vi "SlingPosition.vi"(9 "PhoenixMotorControlDevRef":T1={"DeviceStatus"={"status"=FALSE, "code"=0, "source"=""}, "Type"=enum."PWM", "PWM"={"PWM Channel"=enum."PWM 1", "DeadBand"={"Name"="", "maxPositivePwm"=0, "minPositivePwm"=0, "centerPwm"=0, "maxNegativePwm"=0, "minNegativePwm"=0, "angularRange"=0}}, "CAN"={"Device Number"=0, "SetOutput VI Ref"=variant(enum8{"Percent VBus", "Current", "Speed", "Position", "Voltage"} enum."Percent VBus"), "GetOutput VI Ref"=variant(refnum<k1> refnum), "Enable VI Ref"=variant(dbl 12.0), "Disable VI Ref"=variant(enum8{"Percent VBus", "Speed", "Position", "Slave", "Unchanged / Invalid", "Voltage Compensation", "Current", "Motion Profile"} enum."Percent VBus"), "Data"=variant}, "Invert"=FALSE, "DIO PWM"={"PWM \"Enable\" Channel"=enum."Invalid", "DIOChannel"=enum."Invalid", "PWM Rate"=0.0}}, 11 "SonarSRF04DevRef":T6={"DevStatus"={"status"=FALSE, "code"=0, "source"=""}, "Ping Channel"=enum."Invalid", "Echo Channel"=enum."Invalid", "CntIndex"=enum."Invalid"}) -> (2 "Ready":bool)   [LabVIEW 2017]
uses:
  <vilib>/Rock Robotics/WPI/Ultrasonic/WPI_UltrasonicDeviceRef.ctl
  <vilib>/Rock Robotics/SystemInterfaces/DIO/FPGA_DIOChannel.ctl
  <vilib>/Rock Robotics/SystemInterfaces/Counter/FPGA_CounterCtrSystemIndex.ctl
  <vilib>/Rock Robotics/WPI/MotorControl/WPI_MotorControlDeviceRef.ctl
  <vilib>/Rock Robotics/WPI/MotorControl/WPI_MotorControlType.ctl
  <vilib>/Rock Robotics/SystemInterfaces/DIO/FPGA_DIOPWMChannel.ctl
  <vilib>/Rock Robotics/WPI/PWM/WPI_PWMDeadband.ctl
  Public/Documents/Cross The Road Electronics/Phoenix-LabVIEW/Motor Controller/Controls/CTRE_Phoenix_MotorControl_ControlMode.ctl
  <vilib>/Rock Robotics/WPI/Ultrasonic/WPI_SonarSRF04DigitalGetRange.vi
  Global 1.vi
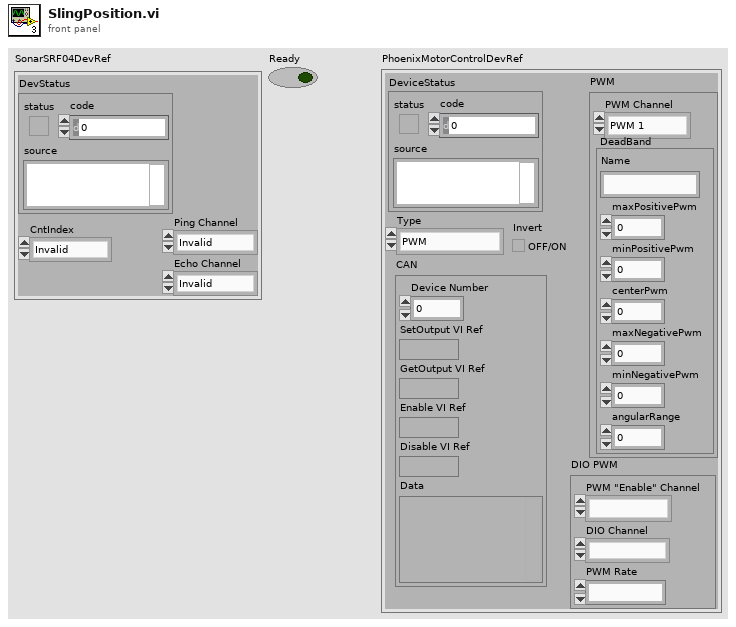
[diagram p1: front panel]
types:
  T1 = typedef "WPI_MotorControlDeviceRef.ctl" = cluster{"DeviceStatus":errorcluster, "Type":T2, "PWM":cluster{"PWM Channel":T3, "DeadBand":T4}, "CAN":cluster{"Device Number":u8, "SetOutput VI Ref":variant, "GetOutput VI Ref":variant, "Enable VI Ref":variant, "Disable VI Ref":variant, "Data":variant}, "Invert":bool, "DIO PWM":cluster{"PWM \"Enable\" Channel":T3, "DIOChannel":T5, "PWM Rate":dbl}}
  T2 = typedef "WPI_MotorControlType.ctl" = enum16{"PWM", "CAN", "DIO PWM"}
  T3 = typedef "FPGA_DIOPWMChannel.ctl" = enum8{"PWM 0", "PWM 1", "PWM 2", "PWM 3", "PWM 4", "PWM 5", "PWM 6", "PWM 7", "PWM 8", "PWM 9", "PWM MXP 0", "PWM MXP 1", "PWM MXP 2", "PWM MXP 3", "PWM MXP 4", "PWM MXP 5", "PWM MXP 6", "PWM MXP 7", "PWM MXP 8", "PWM MXP 9", "Invalid"}
  T4 = typedef "WPI_PWMDeadband.ctl" = cluster{"Name":string, "maxPositivePwm":i32, "minPositivePwm":i32, "centerPwm":i32, "maxNegativePwm":i32, "minNegativePwm":i32, "angularRange":u16}
  T5 = typedef "FPGA_DIOChannel.ctl" = enum8{"DIO 0", "DIO 1", "DIO 2", "DIO 3", "DIO 4", "DIO 5", "DIO 6", "DIO 7", "DIO 8", "DIO 9", "DIO MXP 0", "DIO MXP 1", "DIO MXP 2", "DIO MXP 3", "DIO MXP 4", "DIO MXP 5", "DIO MXP 6", "DIO MXP 7", "DIO MXP 8", "DIO MXP 9", "DIO MXP 10", "DIO MXP 11", "DIO MXP 12", "DIO MXP 13", "DIO MXP 14", "DIO MXP 15", "SPI Port CS1", "SPI Port CS2", "SPI Port CS3", "SPI Port MISO", "SPI Port MOSI", "Invalid"}
  T6 = typedef "WPI_UltrasonicDeviceRef.ctl" = cluster{"DevStatus":errorcluster, "Ping Channel":T5, "Echo Channel":T5, "CntIndex":T7}
  T7 = typedef "FPGA_CounterCtrSystemIndex.ctl" = enum8{"Ctr 0", "Ctr 1", "Ctr 2", "Ctr 3", "Ctr 4", "Ctr 5", "Ctr 6", "Ctr 7", "Invalid"}
  T8 = typedef "CTRE_Phoenix_MotorControl_ControlMode.ctl" = u16
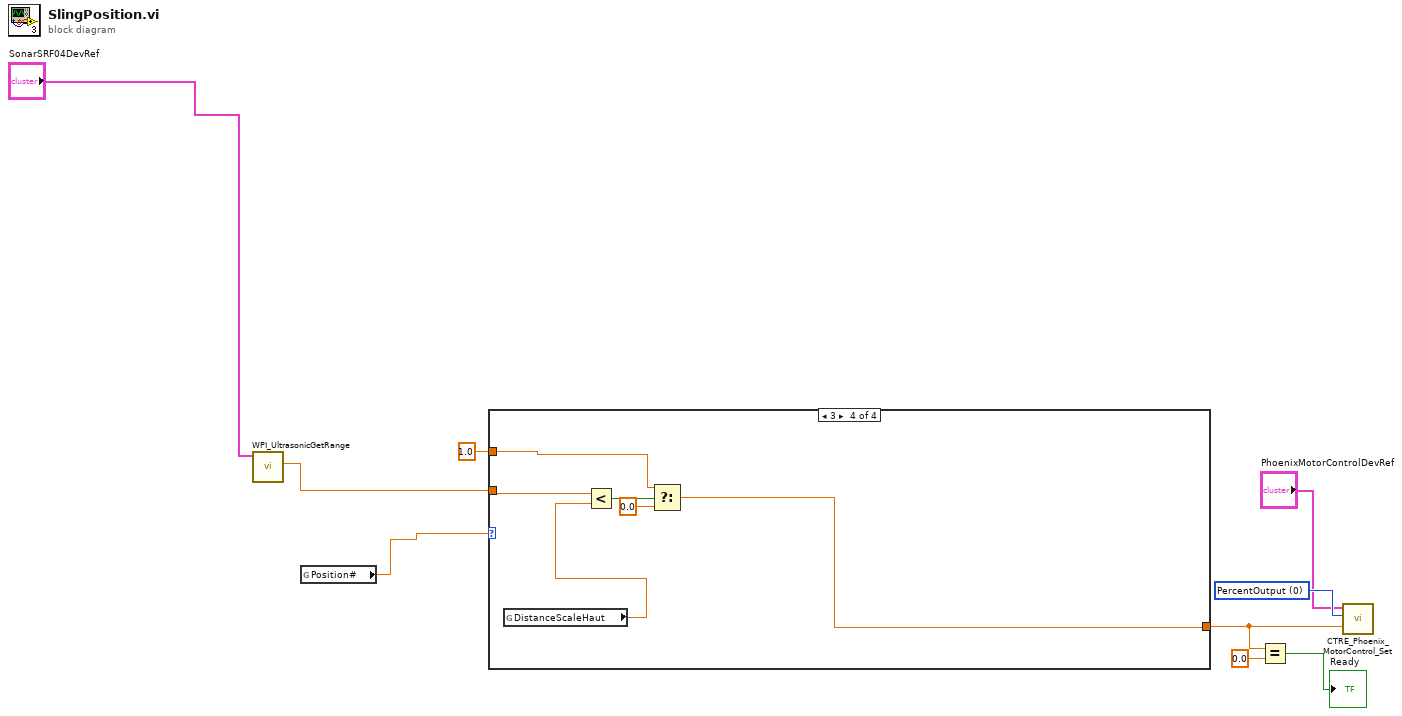
[diagram p0: block diagram]
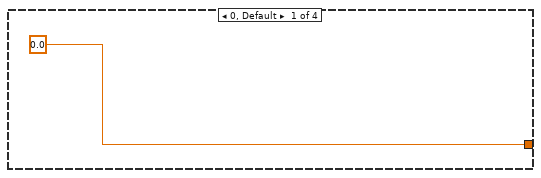
[diagram p2: hidden frame]
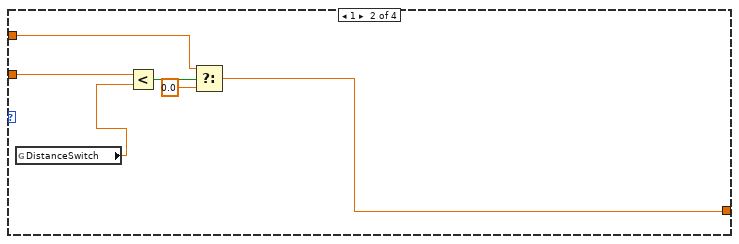
[diagram p3: hidden frame]
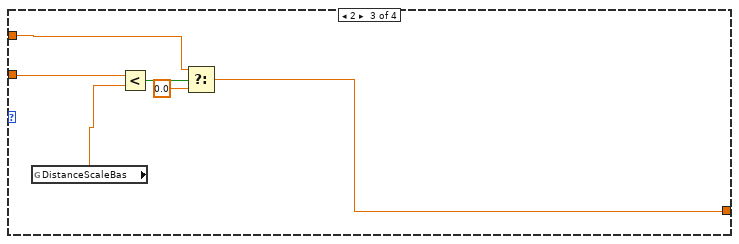
[diagram p4: hidden frame]
diagram:
  w6 = T8 0 items=["PercentOutput"=0, "Position"=1, "Velocity"=2, "Current"=3, "Follower"=5, "MotionProfile"=6, "MotionMagic"=7, "MotionMagicArc"=8, "MotionProfileArc"=10, "Disabled"=15] ("Control Mode")
  n1 = call-poly <vilib>:"WPI_UltrasonicGetRange.vi"("SonarSRF04DevRef"="SonarSRF04DevRef") -> ("Distance"=w9:dbl)  [unwired: 8 in, 2 out]
  n2 = global read "Global 1.vi" "Position#"() -> (w7:dbl)
  n3 = case shown="3" w7 {
    tunnel: [0.0 ("Output") w12 w19 w25] -> w3
    tunnel: w9 -> [_ w16 w18 w24]
    tunnel: 1.0 ("t") -> [_ w14 w20 w26]
    frame 0, Default {
    }
    frame 1 {
      n4 = global read "Global 1.vi" "DistanceSwitch"() -> (w11:dbl)
      n5 = Less?(x=w16, y=w11) -> (x < y?=w15:bool)
      n6 = Select(t=w14, s=w15, f=0.0) -> (s? t:f=w12:dbl)
    }
    frame 2 {
      n7 = global read "Global 1.vi" "DistanceScaleBas"() -> (w17:dbl)
      n8 = Less?(x=w18, y=w17) -> (x < y?=w22:bool)
      n9 = Select(t=w20, s=w22, f=0.0) -> (s? t:f=w19:dbl)
    }
    frame 3 {
      n10 = global read "Global 1.vi" "DistanceScaleHaut"() -> (w23:dbl)
      n11 = Less?(x=w24, y=w23) -> (x < y?=w28:bool)
      n12 = Select(t=w26, s=w28, f=0.0) -> (s? t:f=w25:dbl)
    }
  }
  n13 = Equal?(x=w3, y=0.0) -> (x = y?=→"Ready":bool)
  n14 = call "CTRE_Phoenix_MotorControl_Set.vi"("Output"=w3, "Control Mode"=w6, "PhoenixMotorControlDevRef"="PhoenixMotorControlDevRef") -> ()  [unwired: 7 in, 2 out]
